vi "main_FPGA.vi"() -> ()   [LabVIEW 2015]
uses:
  <vilib>/rvi/Emulation/niFpgaGetClockAttributes.vi
  <vilib>/rvi/Emulation/niFpgaSctlEmulationGetInTimedLoop.vi
  <vilib>/rvi/Emulation/niFpgaEmulationReportErrorSimple.vi
  <vilib>/rvi/Emulation/niFpgaCriticalErrorInLSC.vi
  <vilib>/rvi/eio/common/nirviEmuTemplateMethod_errors.vi
  <vilib>/eio/EIONode/EIONode.xnode
panel:
  in  "NS Extend":bool
  in  "Crosswalk(EW)":bool
  in  "Crosswalk(NS)":bool
  in  "Start":bool
  out "R(NS)":bool
  out "G(NS)":bool
  out "Y(NS)":bool
  out "R(EW)":bool
  out "G(EW)":bool
  out "Y(EW)":bool
  in  "Stop":bool
  out "Time(s)":i16
  in  "PR0":bool
  in  "PR1":bool
  out "Clock Frequency (Hz)":i16
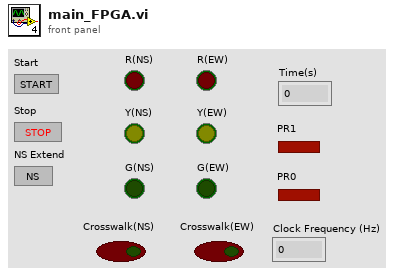
[diagram p1: front panel]
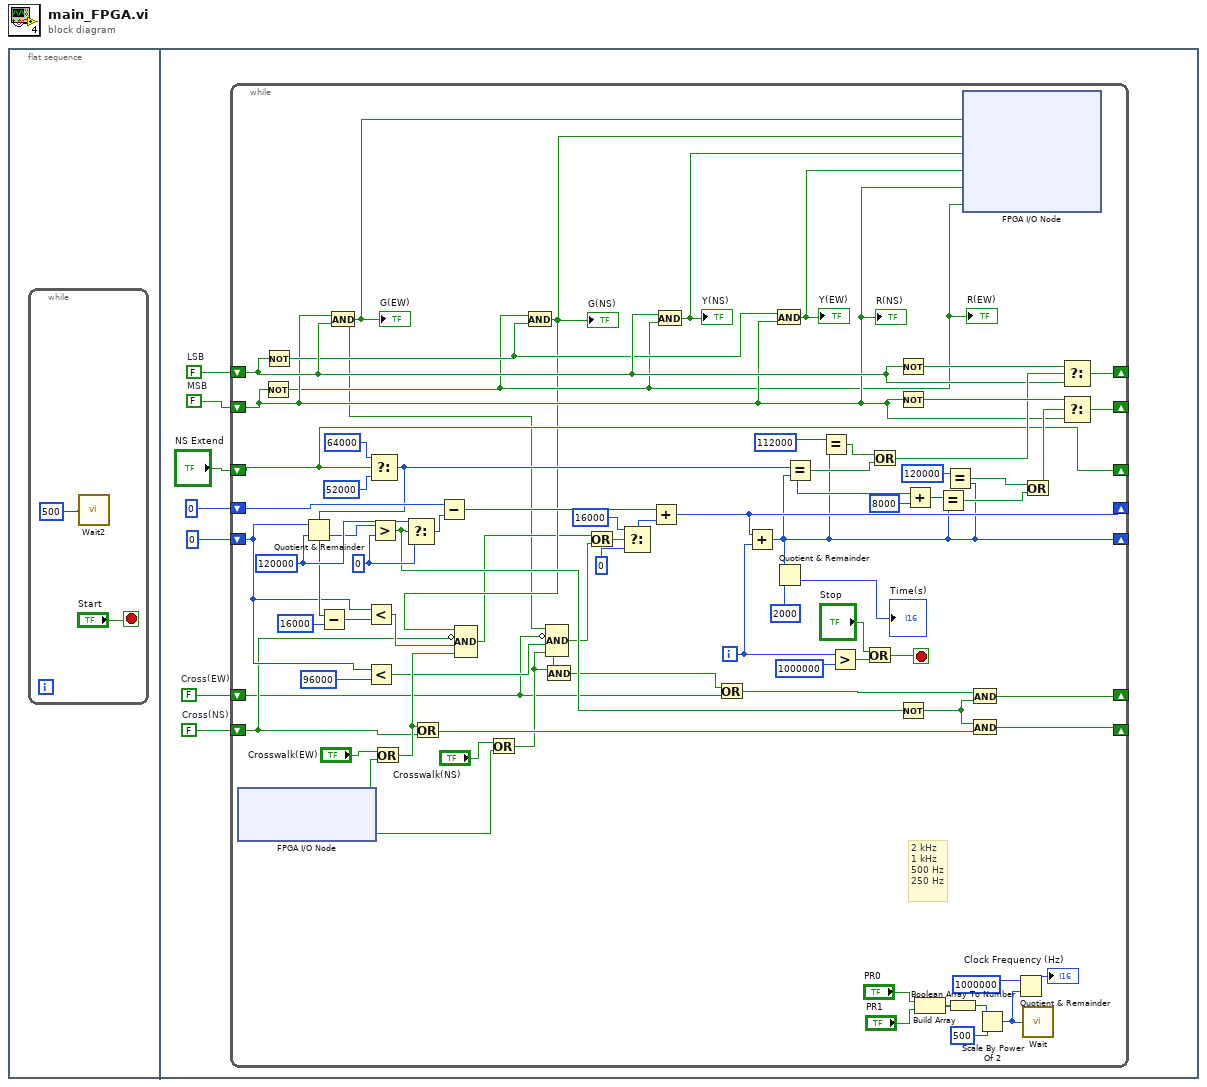
[diagram p0: block diagram]
diagram:
  n1 = flat-sequence {
    frame #0 {
      n2 = while {
        stop <- "Start" stop-if-true
        n3 = call "Wait2"("Count(mSec)"=u32 500) -> ()  [unwired: 1 out]
      }
    }
    frame #1 {
      w4 = FALSE  # Cross(NS)
      w5 = FALSE  # Cross(EW)
      w6 = FALSE  # MSB
      w7 = FALSE  # LSB
      n4 = while {
        shift-right: [w33] -> _
        shift-left: 0 -> [w35]
        shift-right: [w67] -> _
        shift-left: 0 -> [w69]
        shift-right: [w58] -> _
        shift-left: w7 -> [w39]
        shift-right: [w57] -> _
        shift-left: w6 -> [w22]
        shift-right: [w60] -> _
        shift-left: w5 -> [w12]
        shift-right: [w59] -> _
        shift-left: w4 -> [w15]
        shift-right: [w34] -> _
        shift-left: "NS Extend" -> [w34]
        i -> [w73]
        stop <- w77 stop-if-true
        w72 = 0
        w71 = 120000
        # "2 kHz\n1 kHz\n500 Hz\n250 Hz"
        n5 = xnode "FPGA I/O Node"() -> ("ConnectorA/DIO0"=w27:bool, "ConnectorA/DIO1"=w20:bool)  [unwired: 2 in, 2 out]
        n6 = Not(x=w22) -> (.not. x?=w21:bool)
        "R(EW)" <- w21
        n7 = Not(x=w39) -> (.not. x?=w38:bool)
        n8 = Quotient & Remainder(x=w35, y=w71) -> (floor(x/y)=w66:i32)  [unwired: 1 out]
        n9 = And(x=w22, y=w39) -> (x .and. y?=w11:bool)
        "G(EW)" <- w11
        n10 = Less?(x=w35, y=96000) -> (x < y?=w13:bool)
        n11 = Select(t=64000, s=w34, f=52000) -> (s? t:f=w43:i32)
        n12 = Subtract(x=w43, y=16000) -> (x-y=w41:i32)
        n13 = Less?(x=w35, y=w41) -> (x < y?=w18:bool)
        n14 = Greater?(x=w66, y=w72) -> (0:w64:bool)
        n15 = Or(x="Crosswalk(EW)", y=w27) -> (x .or. y?=w19:bool)
        n16 = Select(t=w71, s=w64, f=w72) -> (s? t:f=w70:i32)
        n17 = Or(x=w19, y=w15) -> (x .or. y?=w61:bool)
        n18 = Subtract(x=w69, y=w70) -> (x-y=w68:i32)
        n19 = Or(x="Crosswalk(NS)", y=w20) -> (x .or. y?=w14:bool)
        n20 = And(x=w21, y=w38) -> (x .and. y?=w17:bool)
        "G(NS)" <- w17
        n21 = Compound Arithmetic op=AND(w17, invert w15, w18, w19) -> (w16:bool)
        n22 = And(x=w14, y=w11) -> (x .and. y?=w37:bool)
        n23 = Compound Arithmetic op=AND(w11, invert w12, w13, w14) -> (w10:bool)
        n24 = Or(x=w16, y=w10) -> (x .or. y?=w65:bool)
        n25 = Select(t=16000, s=w65, f=0) -> (s? t:f=w74:i32)
        n26 = Add(x=w68, y=w74) -> (x+y=w67:i32)
        n27 = And(x=w39, y=w21) -> (x .and. y?=w24:bool)
        "Y(NS)" <- w24
        n28 = Or(x=w37, y=w12) -> (x .or. y?=w62:bool)
        n29 = Add(x=w67, y=w73) -> (x+y=w33:i32)
        n30 = And(x=w38, y=w22) -> (x .and. y?=w23:bool)
        "Y(EW)" <- w23
        n31 = Quotient & Remainder(x=w33, y=2000) -> (floor(x/y)=→"Time(s)":i32)  [unwired: 1 out]
        n32 = Equal?(x=w43, y=w33) -> (x = y?=w50:bool)
        n33 = Equal?(x=112000, y=w33) -> (x = y?=w51:bool)
        n34 = Greater?(x=w73, y=1000000) -> (0:w79:bool)
        n35 = Or(x="Stop", y=w79) -> (x .or. y?=w77:bool)
        n36 = Or(x=w51, y=w50) -> (x .or. y?=w49:bool)
        n37 = Not(x=w39) -> (.not. x?=w56:bool)
        n38 = Not(x=w22) -> (.not. x?=w55:bool)
        n39 = Not(x=w64) -> (.not. x?=w63:bool)
        n40 = Add(x=w43, y=8000) -> (x+y=w36:i32)
        n41 = Build Array("PR0", "PR1") -> (w82:bool[])
        n42 = Equal?(x=w36, y=w33) -> (x = y?=w47:bool)
        n43 = Equal?(x=120000, y=w33) -> (x = y?=w48:bool)
        n44 = Boolean Array To Number(Boolean array=w82) -> (number=w81:u32)
        n45 = xnode "FPGA I/O Node"("ConnectorA/DIO4"=w11, "ConnectorA/DIO7"=w17, "ConnectorA/DIO6"=w24, "ConnectorA/DIO3"=w23, "ConnectorA/DIO5"=w22, "ConnectorA/DIO2"=w21) -> ()  [unwired: 6 in, 6 out]
        n46 = And(x=w62, y=w63) -> (x .and. y?=w60:bool)
        n47 = And(x=w63, y=w61) -> (x .and. y?=w59:bool)
        n48 = Scale By Power Of 2(n=w81, x=u32 500 ("Count(mSec)")) -> (x*2^n=w29:u32)
        n49 = Quotient & Remainder(x=1000000, y=w29) -> (floor(x/y)=→"Clock Frequency (Hz)":u32)  [unwired: 1 out]
        n50 = Or(x=w48, y=w47) -> (x .or. y?=w44:bool)
        n51 = call "Wait"("Count(uSec)"=w29) -> ()  [unwired: 1 out]
        n52 = Select(t=w56, s=w49, f=w39) -> (s? t:f=w58:bool)
        n53 = Select(t=w55, s=w44, f=w22) -> (s? t:f=w57:bool)
        "R(NS)" <- w22
      }
    }
  }
